vi "UnpackFieldsFromAny.vi"(8 "error in":errorcluster, 11 "Any":T1) -> (0 "error out":errorcluster, 3 "Fields Ref Out":T2)   [LabVIEW 2019, in "grpc-lvsupport.lvlib"]
uses:
  grpc-lvsupport.lvlib
  Shared/grpcId.ctl
  Shared/Any.ctl
  <vilib>/AdvancedString/1D String Array to Delimited String.vi
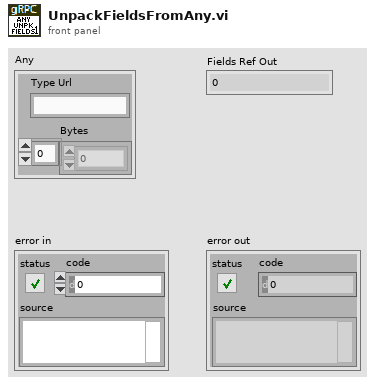
[diagram p1: front panel]
types:
  T1 = typedef "grpc-lvsupport.lvlib/Any.ctl" = cluster{"Type Url":string, "Bytes":u8[]}
  T2 = typedef "grpc-lvsupport.lvlib/grpcId.ctl" = u64
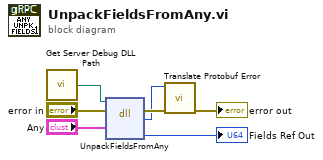
[diagram p0: block diagram]
diagram:
  n1 = call "Get Server Debug DLL Path.vi"() -> ("Server Debug DLL Path"=w5:path)
  n2 = dll-call lib="?" fn="UnpackFieldsFromAny"(path in=w5, error in="error in", "any"="Any") -> (error out=w6:errorcluster, "return type"=w1:i32, "elementRef"=→"Fields Ref Out":u64)  [unwired: 3 in, 1 out]
  n3 = call "Translate Protobuf Error.vi"("error in"=w6, "Error Code"=w1) -> ("error out"=→"error out":errorcluster)  [unwired: 9 in]
